vi "compute_center_of_mass.vi"(8 "end":i32=-1, 9 "start":i32=-1, 11 "array":i16[](array[numeric])) -> (3 "center of  'mass'":u16)   [LabVIEW 2012]
uses:
  <vilib>/NXT/Dual Mode Library/prims/addArrayElements_int.vi
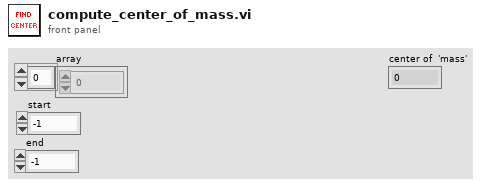
[diagram p1: front panel]
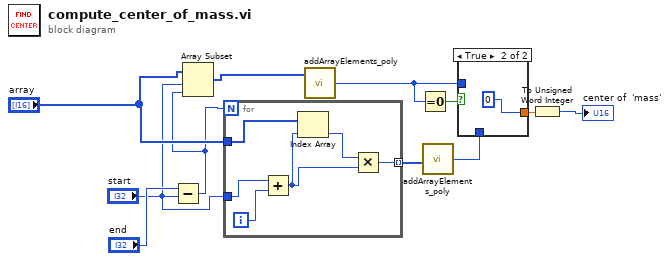
[diagram p0: block diagram]
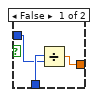
[diagram p2: hidden frame]
diagram:
  n1 = Subtract(x="end", y="start") -> (x-y=w3:i32)
  n2 = Array Subset(array="array", index="start", length=w3) -> (w5:i16[])
  n3 = for {
    N: w3 -> [_]
    tunnel: "start" -> [w16]
    tunnel: "array" -> [w15]
    tunnel: [w12] -> w10 mode=indexing
    i -> [w17]
    n4 = Add(x=w16, y=w17) -> (x+y=w14:i32)
    n5 = Index Array(array=w15, index=w14) -> (element=w13:i16)
    n6 = Multiply(x=w13, y=w14) -> (x*y=w12:i32)
  }
  n7 = call-poly <vilib>:"addArrayElements_poly.vi"("Numeric Array"=w5) -> ("Sum"=w2:i32)
  n8 = Equal To 0?(x=w2) -> (x = 0?=w1:bool)
  n9 = call-poly <vilib>:"addArrayElements_poly.vi"("Numeric Array"=w10) -> ("Sum"=w9:i32)
  n10 = case shown="True" w1 {
    tunnel: w9 -> [w20 _]
    tunnel: w2 -> [w19 _]
    tunnel: [w18 0] -> w8
    frame False {
      n11 = Divide(x=w20, y=w19) -> (x/y=w18:dbl)
    }
    frame True {
    }
  }
  n12 = To Unsigned Word Integer(number=w8) -> (unsigned 16bit integer=→"center of  'mass'":u16)
